vi "mul gpos.vi"() -> ()   [LabVIEW 2020]
uses:
  <vilib>/Analysis/Matrix/Datatypes/RealMatrix.ctl
  <vilib>/Analysis/Matrix/Numeric/Conversions/Array To Matrix - RA.vi
  <vilib>/Analysis/Matrix/Numeric/Conversions/Array To Matrix - RA2.vi
  <vilib>/Analysis/Matrix/Numeric/Multiply/Multiply - RM,RM.vi
  <vilib>/Utility/file.llb/Write Delimited Spreadsheet (I64).vi
  <vilib>/Analysis/Matrix/NI_Matrix.lvlib
panel:
  out "overall time":u32
  in  "timing data out":path
  out "product":T1
  in  "vector size":i32=20
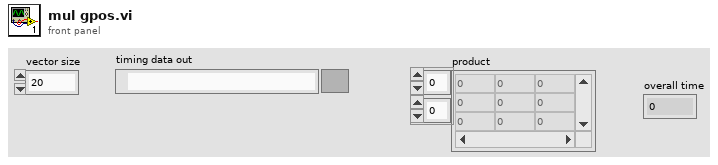
[diagram p1: front panel]
types:
  T1 = typedef "NI_Matrix.lvlib/RealMatrix.ctl" = dbl[][]
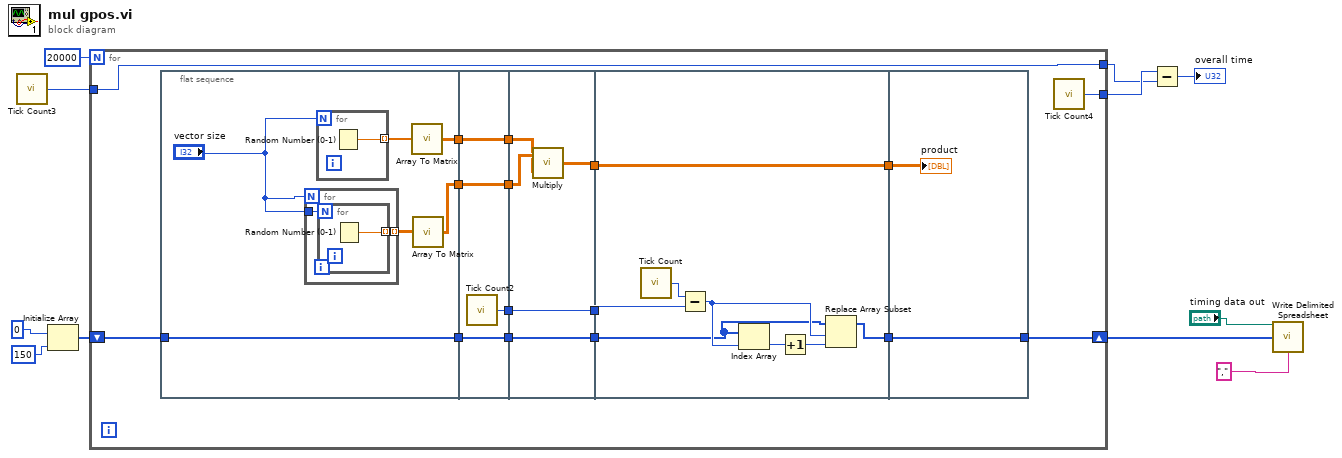
[diagram p0: block diagram]
diagram:
  n1 = call "Tick Count3"() -> ("Tick Count(uSec)"=w4:u32)
  n2 = Initialize Array(0, 150) -> (w8:i32[])
  n3 = for {
    N: 20000 -> [_]
    shift-right: [w14] -> w5
    shift-left: w8 -> [w16]
    tunnel: [w13] -> w2
    tunnel: w4 -> [w13]
    tunnel: [w12] -> w3
    n4 = flat-sequence {
      tunnel: [w32] -> w27
      tunnel: [w30] -> w21
      tunnel: [w28] -> w17
      tunnel: w16 -> [w28]
      tunnel: w27 -> [w41]
      tunnel: [w41] -> w26
      tunnel: [w40] -> w25
      tunnel: [w39] -> w22
      tunnel: w21 -> [w39]
      tunnel: [w38] -> w18
      tunnel: w17 -> [w38]
      tunnel: w26 -> [w44]
      tunnel: w25 -> [w46]
      tunnel: [w46] -> w24
      tunnel: [w43] -> w23
      tunnel: w22 -> [w45]
      tunnel: [w42] -> w19
      tunnel: w18 -> [w42]
      tunnel: w23 -> [w52]
      tunnel: w24 -> [w53]
      tunnel: [w52] -> w20
      tunnel: w19 -> [w48]
      tunnel: [w47] -> w15
      tunnel: w20 -> [w56]
      tunnel: w15 -> [w55]
      tunnel: [w55] -> w14
      frame #0 {
        n5 = for {
          N: "vector size" -> [_]
          tunnel: [w35] -> w31 mode=indexing
          tunnel: "vector size" -> [w34]
          n6 = for {
            N: w34 -> [_]
            tunnel: [w36] -> w35 mode=indexing
            n7 = Random Number (0-1)() -> (number: 0 to 1=w36:dbl)
          }
        }
        n8 = for {
          N: "vector size" -> [_]
          tunnel: [w37] -> w33 mode=indexing
          n9 = Random Number (0-1)() -> (number: 0 to 1=w37:dbl)
        }
        n10 = call-poly <vilib>:"Array To Matrix.vi"("Real 1D Array"=w33) -> ("Real Matrix (Column Vector)"=w32:T1)
        n11 = call-poly <vilib>:"Array To Matrix.vi"("Real 2D Array"=w31) -> ("Real Matrix"=w30:T1)
      }
      frame #1 {
        n12 = call "Tick Count2"() -> ("Tick Count(uSec)"=w40:u32)
      }
      frame #2 {
        n13 = call-poly <vilib>:"Multiply.vi"("Real Matrix B"=w44, "Real Matrix A"=w45) -> ("A * B"=w43:T1)
      }
      frame #3 {
        n14 = call "Tick Count"() -> ("Tick Count(uSec)"=w54:u32)
        n15 = Subtract(x=w54, y=w53) -> (x-y=w49:u32)
        n16 = Index Array(array=w48, index=w49) -> (element=w50:i32)
        n17 = Increment(x=w50) -> (x+1=w51:i32)
        n18 = Replace Array Subset(array=w48, new element=w51, index=w49) -> (w47:i32[])
      }
      frame #4 {
        "product" <- w56
      }
    }
    n19 = call "Tick Count4"() -> ("Tick Count(uSec)"=w12:u32)
  }
  n20 = Subtract(x=w3, y=w2) -> (x-y=→"overall time":u32)
  n21 = call-poly <vilib>:"Write Delimited Spreadsheet.vi"("file path (dialog if empty)"="timing data out", "1D data"=w5, "delimiter (\\t)"=",") -> ()  [unwired: 11 in, 2 out]
